vi "DSP_init_fast_sweep.vi"(1 "Sample count":u32, 2 "ramp?":bool, 3 "Inst info":T1) -> ()   [LabVIEW 2013]
panel:
  out "error out":errorcluster
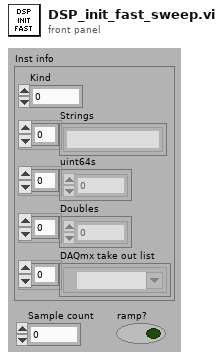
[diagram p1: front panel]
types:
  T1 = cluster{"Kind":u16, "Strings":string[], "uint64s":u64[], "Doubles":dbl[], "DAQmx take out list":refnum<k21>[]}
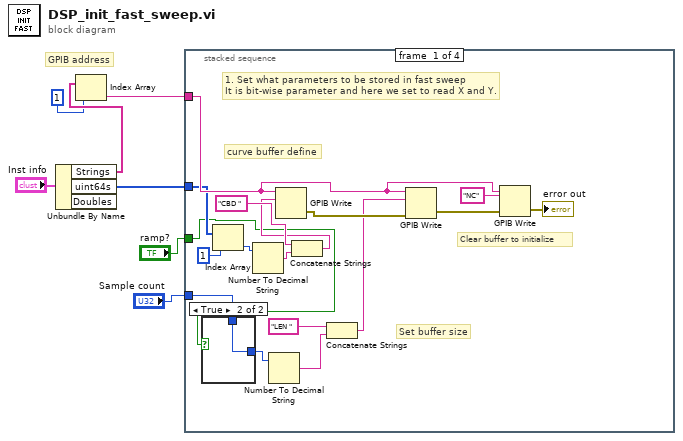
[diagram p0: block diagram]
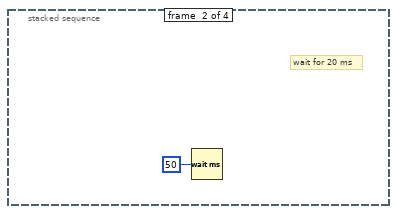
[diagram p3: hidden frame]
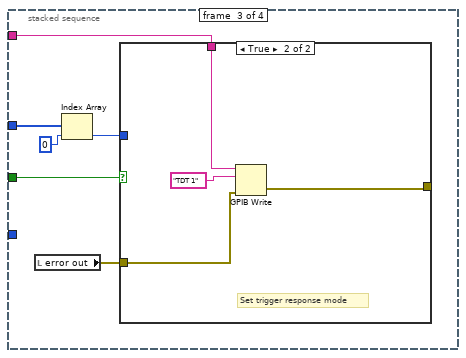
[diagram p4: hidden frame]
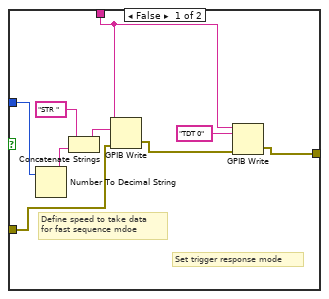
[diagram p5: hidden frame]
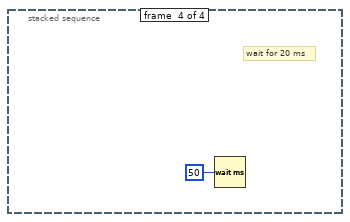
[diagram p6: hidden frame]
diagram:
  # "GPIB address"
  n1 = Unbundle By Name("Inst info") -> ("Strings"=w6:string[], "uint64s"=w1:u64[])  [unwired: 1 out]
  n2 = Index Array(array=w6, index=1) -> (element=w4:string)
  n3 = stacked-sequence {
    tunnel: w4 -> [w18 _ w28 _]
    tunnel: "Sample count" -> [w9 _ _ _]
    tunnel: "ramp?" -> [w10 _ w33 _]
    tunnel: w1 -> [w16 _ w31 _]
    frame #0 {
      # "curve buffer define"
      # "Clear buffer to initialize"
      # "Set buffer size"
      # "1. Set what parameters to be stored in fast sweep\nIt is bit-wise parameter and here we set to read X and Y."
      n4 = case shown="True" w10 {
        tunnel: w9 -> [w25 w26]
        tunnel: [w25 w26] -> w8
        frame False {
        }
        frame True {
        }
      }
      n5 = Index Array(array=w16, index=1) -> (element=w14:u64)
      n6 = Number To Decimal String(number=w14) -> (decimal integer string=w13:string)  [unwired: 1 in]
      n7 = Number To Decimal String(number=w8) -> (decimal integer string=w22:string)  [unwired: 1 in]
      n8 = Concatenate Strings("CBD ", w13) -> (w11:string)
      n9 = GPIB Write(0:w18, 1:w11) -> (6:w24:errorcluster)  [unwired: 3 in, 1 out]
      n10 = Concatenate Strings("LEN ", w22) -> (w21:string)
      n11 = GPIB Write(0:w18, 1:w21, 3:w24) -> (6:w20:errorcluster)  [unwired: 2 in, 1 out]
      n12 = GPIB Write(0:w18, 1:"NC", 3:w20) -> (6:→"error out":errorcluster)  [unwired: 2 in, 1 out]
    }
    frame #1 {
      # "wait for 20 ms"
      n13 = Wait (ms)(milliseconds to wait=50) -> ()  [unwired: 1 out]
    }
    frame #2 {
      n14 = local read "error out"() -> (w32:errorcluster)
      n15 = Index Array(array=w31, index=0) -> (element=w29:u64)
      n16 = case shown="True" w33 {
        tunnel: w28 -> [w41 w46]
        tunnel: w32 -> [w36 w44]
        tunnel: w29 -> [w38 _]
        tunnel: [w34 w43] -> _
        frame False {
          # "Define speed to take data\nfor fast sequence mdoe"
          # "Set trigger response mode"
          n17 = Number To Decimal String(number=w38) -> (decimal integer string=w37:string)  [unwired: 1 in]
          n18 = Concatenate Strings("STR ", w37) -> (w39:string)
          n19 = GPIB Write(0:w41, 1:w39, 3:w36) -> (6:w35:errorcluster)  [unwired: 2 in, 1 out]
          n20 = GPIB Write(0:w41, 1:"TDT 0", 3:w35) -> (6:w34:errorcluster)  [unwired: 2 in, 1 out]
        }
        frame True {
          # "Set trigger response mode"
          n21 = GPIB Write(0:w46, 1:"TDT 1", 3:w44) -> (6:w43:errorcluster)  [unwired: 2 in, 1 out]
        }
      }
    }
    frame #3 {
      # "wait for 20 ms"
      n22 = Wait (ms)(milliseconds to wait=50) -> ()  [unwired: 1 out]
    }
  }
